vi "selected_cities_to_title_string.vi"(8 "error in":errorcluster, 11 "selected_cities":bool[](array[boolean])) -> (0 "error out":errorcluster, 3 "title_string":string)   [LabVIEW 2018]
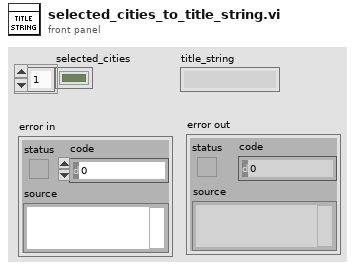
[diagram p1: front panel]
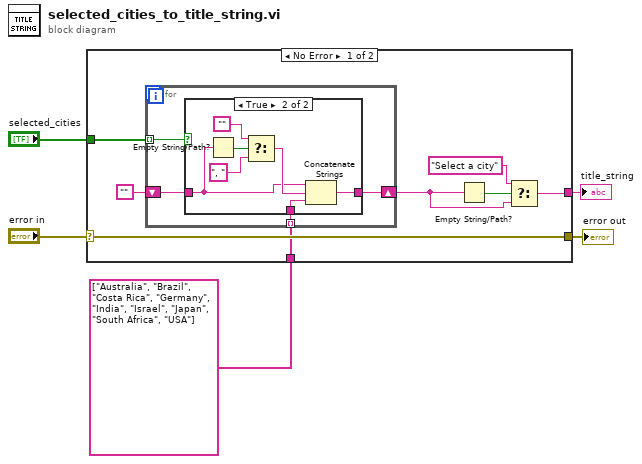
[diagram p0: block diagram]
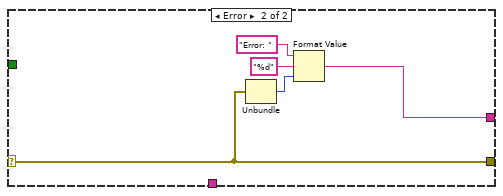
[diagram p3: hidden frame]
diagram:
  n1 = case shown="No Error" "error in" {
    selector: "error in" -> [w13 w29]
    tunnel: [w13 w29] -> w4
    tunnel: "selected_cities" -> [w12 _]
    tunnel: [w7 w26] -> w2
    tunnel: string[] ["Australia", "Brazil", "Costa Rica", "Germany", "India", "Israel", "Japan", "South Africa", "USA"] -> [w6 _]
    frame No Error {
      n2 = for {
        tunnel: w12 -> [w17] mode=indexing
        shift-right: [w15] -> w9
        shift-left: "" -> [w16]
        tunnel: w6 -> [w14] mode=indexing
        n3 = case shown="True" w17 {
          tunnel: w16 -> [w18 w19]
          tunnel: [w18 w25] -> w15
          tunnel: w14 -> [_ w20]
          frame False {
          }
          frame True {
            n4 = Empty String/Path?(string/path=w19) -> (empty?=w24:bool)
            n5 = Select(t="", s=w24, f=", ") -> (s? t:f=w22:string)
            n6 = Concatenate Strings(w19, w22, w20) -> (w25:string)
          }
        }
      }
      n7 = Empty String/Path?(string/path=w9) -> (empty?=w10:bool)
      n8 = Select(t="Select a city" ("title"), s=w10, f=w9) -> (s? t:f=w7:string)
    }
    frame Error {
      n9 = Unbundle(w29) -> ("code"=w28:i32)  [unwired: 2 out]
      n10 = Format Value(string ("")="Error: ", format string="%d", value (0)=w28) -> (output string=w26:string)
    }
  }
  "title_string" <- w2
  "error out" <- w4
